vi "Init Transition.vi"(7 "VolatusAPI":refnum<class "VolatusAPI.lvclass">, 8 "error in (no error)":refnum<class "MultiErrors.lvclass">, 10 "Transition Config":refnum<class "Transition Config.lvclass">, 11 "Transition in":refnum<class "Transition.lvclass">) -> (0 "error out":refnum<class "MultiErrors.lvclass">, 3 "Transition out":refnum<class "Transition.lvclass">)   [LabVIEW 2020, in "VolatusSeq.lvlib" / "Transition.lvclass"]
uses:
  Transition.lvclass
  Volatus/VolatusAPI/VolatusAPI.lvclass
  VolatusSeqConfig/Transition Config/Transition Config.lvclass
  Transition.lvclass/Transition.ctl
  Volatus/MultiErrors/MultiErrors.lvclass
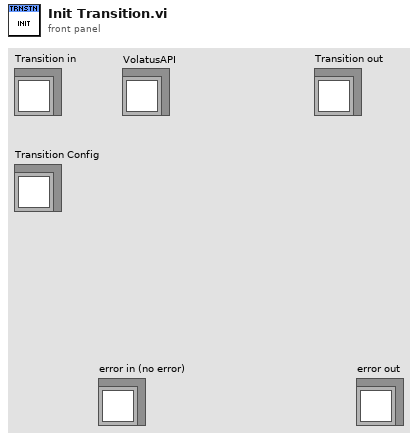
[diagram p1: front panel]
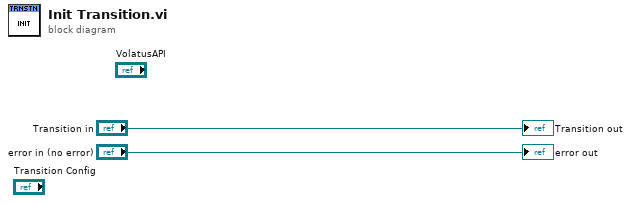
[diagram p0: block diagram]
diagram:
  "error out" <- "error in (no error)"
  "Transition out" <- "Transition in"
